vi "Process Analog Configuration.vi"(7 "PMU Name":string, 11 "Analog Configuration In":T1) -> (1 "Analog Channel Types":u8[](array[numeric]), 2 "Analog Channel Names":string[](array[string]), 3 "Analog Configuration Out":T2(array[cluster]))   [LabVIEW 2013, in "PMU Recorder Light.lvlib" / "Phasor Data Concentrator.lvclass"]
uses:
  Phasor Data Concentrator.lvclass
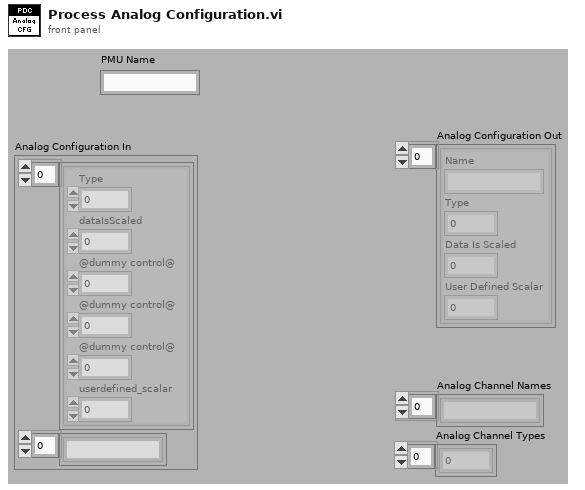
[diagram p1: front panel]
types:
  T1 = cluster{cluster{"Type":i32, "dataIsScaled":u8, "@dummy control@":i8, "@dummy control@":i8, "@dummy control@":i8, "userdefined_scalar":sgl}[], string[]}
  T2 = cluster{"Name":string, "Type":i32, "Data Is Scaled":u8, "User Defined Scalar":sgl}[]
  T3 = cluster{"Type":i32, "dataIsScaled":u8, "@dummy control@":i8, "@dummy control@":i8, "@dummy control@":i8, "userdefined_scalar":sgl}[]
  T4 = cluster{"Name":string, "Type":i32, "Data Is Scaled":u8, "User Defined Scalar":sgl}
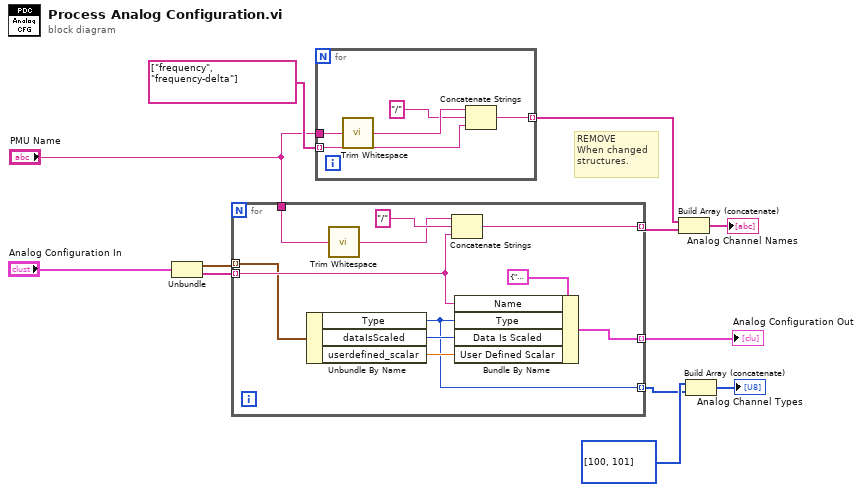
[diagram p0: block diagram]
diagram:
  # "REMOVE\nWhen changed\nstructures."
  n1 = Unbundle("Analog Configuration In") -> (w11:T3, w10:string[])
  n2 = for {
    tunnel: [w22] -> w6 mode=indexing
    tunnel: "PMU Name" -> [w20]
    tunnel: w10 -> [w19] mode=indexing
    tunnel: w11 -> [w18] mode=indexing
    tunnel: [w15] -> w12 mode=indexing
    tunnel: [w13] -> w2 mode=indexing
    n3 = Unbundle By Name(w18) -> ("Type"=w13:i32, "dataIsScaled"=w17:u8, "userdefined_scalar"=w16:sgl)
    n4 = call <vilib>:"Trim Whitespace.vi"("string"=w20) -> ("trimmed string"=w21:string)  [unwired: 1 in]
    n5 = Concatenate Strings(w21, "/" ("string"), w19) -> (w22:string)
    n6 = Bundle By Name(cluster=T4 {"Name"="", "Type"=0, "Data Is Scaled"=0, "User Defined Scalar"=0.0} ("Analog Configuration"), "Name"=w19, "Type"=w13, "Data Is Scaled"=w17, "User Defined Scalar"=w16) -> (w15:T4)
  }
  "Analog Configuration Out" <- w12
  n7 = for {
    tunnel: string[] ["frequency", "frequency-delta"] -> [w26] mode=indexing
    tunnel: "PMU Name" -> [w25]
    tunnel: [w24] -> w5 mode=indexing
    n8 = call <vilib>:"Trim Whitespace.vi"("string"=w25) -> ("trimmed string"=w28:string)  [unwired: 1 in]
    n9 = Concatenate Strings(w28, "/" ("string"), w26) -> (w24:string)
  }
  n10 = Build Array (concatenate)(w5, w6) -> (→"Analog Channel Names":string[])
  n11 = Build Array (concatenate)(i32[] [100, 101], w2) -> (→"Analog Channel Types":i32[])
